vi "AdjustSpeaker.vi"(1 "Input Signal":refnum<vi>, 4 "Terminate":refnum<vi>, 5 "Peiker_Stepped Sweep Settings":T3={"Input Settings"={"IEPE min time to settle [s]"=0.0, "Responce Channel Settings"={"DSA response channel settings"={"coupling"=10045, "enable IEPE excitation"=FALSE, "IEPE current [mA]"=4.0}, "response channel info"={"sensor sensitivity"=200.0, "engineering units"=2, "dB reference"=2e-05, "custom label"="EU", "weighting filter"=0, "pregain"=0.0}, "AI response settings"={"response channel"="SOUNDACQ/ai1", "max value [V]"=10.0, "min value [V]"=-10.0, "terminal configuration"=-1}}, "Stimulus Channel Settings"={"AI stimulus settings"={"stimulus channel"="SOUNDACQ/ai0", "max value [V]"=10.0, "min value [V]"=-10.0, "terminal configuration"=-1}, "DSA stimulus channel settings"={"coupling"=10045, "enable IEPE excitation"=TRUE, "IEPE current [mA]"=4.0}, "stimulus channel info"={"sensor sensitivity"=11.4, "engineering units"=2, "dB reference"=2e-05, "custom label"="EU", "weighting filter"=0, "pregain"=0.0}}}, "Output Settings"={"AO source settings"={"excitation channel"="SOUNDACQ/ao0", "max value [V]"=10.0, "min value [V]"=-10.0, "terminal configuration"=-1}}} {"Output Settings"."AO source settings"."terminal configuration" items=["Default"=-1, "RSE"=10083, "Differential"=10106, "Pseudodifferential"=12529]; "Output Settings"."AO source settings"."min value [V]" format="%0.2f"; "Output Settings"."AO source settings"."max value [V]" format="%0.2f"; "Input Settings"."Stimulus Channel Settings"."stimulus channel info"."pregain" format="%.2f"; "Input Settings"."Stimulus Channel Settings"."stimulus channel info"."weighting filter" items=["Linear", "A-weighting", "B-weighting", "C-weighting", "ITU-R 468-4", "Dolby", "CCITT", "C-message", "Wb", "Wc", "Wd", "We", "Wf", "Wh", "Wj", "Wk", "Wm", "AES17 20 kHz lowpass", "AES17 40 kHz lowpass", "AES17 20 kHz highpass", "AES17 40 kHz highpass"]; "Input Settings"."Stimulus Channel Settings"."stimulus channel info"."dB reference" format="%^.1e"; "Input Settings"."Stimulus Channel Settings"."stimulus channel info"."engineering units" items=["custom..."=0, "V"=1, "A"=21, "C"=30, "pC"=31, "s"=32, "-"=29, "Pa"=2, "N"=20, "g"=3, "m/s^2"=4, "m/s"=5, "m"=6, "mm/s"=12, "mm"=13, "micron/s"=14, "micron"=15, "in/s^2"=7, "in/s"=8, "in"=9, "mil/s"=10, "mil"=11, "rad/s^2"=16, "rad/s"=17, "rad"=18, "deg/s^2"=26, "deg/s"=27, "deg"=28, "RPM"=22, "cycle/s^2"=23, "Hz"=24, "cycle"=25, "strain"=19]; "Input Settings"."Stimulus Channel Settings"."stimulus channel info"."sensor sensitivity" format="%#_5f"; "Input Settings"."Stimulus Channel Settings"."DSA stimulus channel settings"."IEPE current [mA]" format="%.1f"; "Input Settings"."Stimulus Channel Settings"."DSA stimulus channel settings"."coupling" items=["AC"=10045, "DC"=10050, "GND"=10066]; "Input Settings"."Stimulus Channel Settings"."AI stimulus settings"."terminal configuration" items=["Default"=-1, "RSE"=10083, "NRSE"=10078, "Differential"=10106, "Pseudodifferential"=12529]; "Input Settings"."Stimulus Channel Settings"."AI stimulus settings"."min value [V]" format="%.2f"; "Input Settings"."Stimulus Channel Settings"."AI stimulus settings"."max value [V]" format="%.2f"; "Input Settings"."Responce Channel Settings"."AI response settings"."terminal configuration" items=["Default"=-1, "RSE"=10083, "NRSE"=10078, "Differential"=10106, "Pseudodifferential"=12529]; "Input Settings"."Responce Channel Settings"."AI response settings"."min value [V]" format="%.2f"; "Input Settings"."Responce Channel Settings"."AI response settings"."max value [V]" format="%.2f"; "Input Settings"."Responce Channel Settings"."response channel info"."pregain" format="%.2f"; "Input Settings"."Responce Channel Settings"."response channel info"."weighting filter" items=["Linear", "A-weighting", "B-weighting", "C-weighting", "ITU-R 468-4", "Dolby", "CCITT", "C-message", "Wb", "Wc", "Wd", "We", "Wf", "Wh", "Wj", "Wk", "Wm", "AES17 20 kHz lowpass", "AES17 40 kHz lowpass", "AES17 20 kHz highpass", "AES17 40 kHz highpass"]; "Input Settings"."Responce Channel Settings"."response channel info"."dB reference" format="%^.1e"; "Input Settings"."Responce Channel Settings"."response channel info"."engineering units" items=["custom..."=0, "V"=1, "A"=21, "C"=30, "pC"=31, "s"=32, "-"=29, "Pa"=2, "N"=20, "g"=3, "m/s^2"=4, "m/s"=5, "m"=6, "mm/s"=12, "mm"=13, "micron/s"=14, "micron"=15, "in/s^2"=7, "in/s"=8, "in"=9, "mil/s"=10, "mil"=11, "rad/s^2"=16, "rad/s"=17, "rad"=18, "deg/s^2"=26, "deg/s"=27, "deg"=28, "RPM"=22, "cycle/s^2"=23, "Hz"=24, "cycle"=25, "strain"=19]; "Input Settings"."Responce Channel Settings"."response channel info"."sensor sensitivity" format="%#_5f"; "Input Settings"."Responce Channel Settings"."DSA response channel settings"."IEPE current [mA]" format="%.1f"; "Input Settings"."Responce Channel Settings"."DSA response channel settings"."coupling" items=["AC"=10045, "DC"=10050, "GND"=10066]; "Input Settings"."IEPE min time to settle [s]" format="%.1f"}, 6 "Fundamental Amplitude 2":refnum<vi>, 7 "CalSettings":T1={"SollPegel[dBSPL]"=114, "maxDeviationRef[dB]"=2.0, "maxDeviation[dB]"=2.0, "maxRuns"=20, "RefFrequency[Hz]"=1000, "Wait[ms]"=0} {"maxDeviation[dB]" format="%.2f"; "maxDeviationRef[dB]" format="%.2f"}, 8 "error in":errorcluster, 9 "integration time":T9={"integration time [s]"=0.015599999576807022, "integration cycles"=5} {"integration cycles" min=2; "integration time [s]" format="%.2p"}, 10 "settling time":T8={"settle time [s]"=0.015599999576807022, "settle cycles"=5} {"settle time [s]" format="%.2p"}, 11 "Frequency List":T2(array[cluster])) -> (0 "error out":errorcluster, 2 "magnitude":dbl[](array[numeric]), 3 "correctedFreqList":T2(array[cluster]))   [LabVIEW 2018]
uses:
  Peiker_Stepped Sweep Settings.ctl
  <vilib>/addons/_NISVFA/_Shared subVIs/Controls/svc_DSA Channel Settings.ctl
  <vilib>/addons/_NISVFA/_Shared subVIs/Controls/svc_Channel Info.ctl
  <vilib>/addons/_NISVFA/_Shared subVIs/Controls/svc_Engineering Units Text Ring.ctl
  <vilib>/addons/_NISVFA/_Shared subVIs/Controls/svc_Weighting Filter Text Ring.ctl
panel:
  out "error out 2":errorcluster
  out "max value":dbl
  out "min value":dbl
  out "RefValue":dbl
  in  "CalTablePath":path=path "D:/PRUEF/MIC_EOL_TS2016/Sourcecode/ProjectSourcecode/Config Files/calibrationResults.txt"
  out "runs":i32
  # "Input Parameters"
  # "Output Parameters"
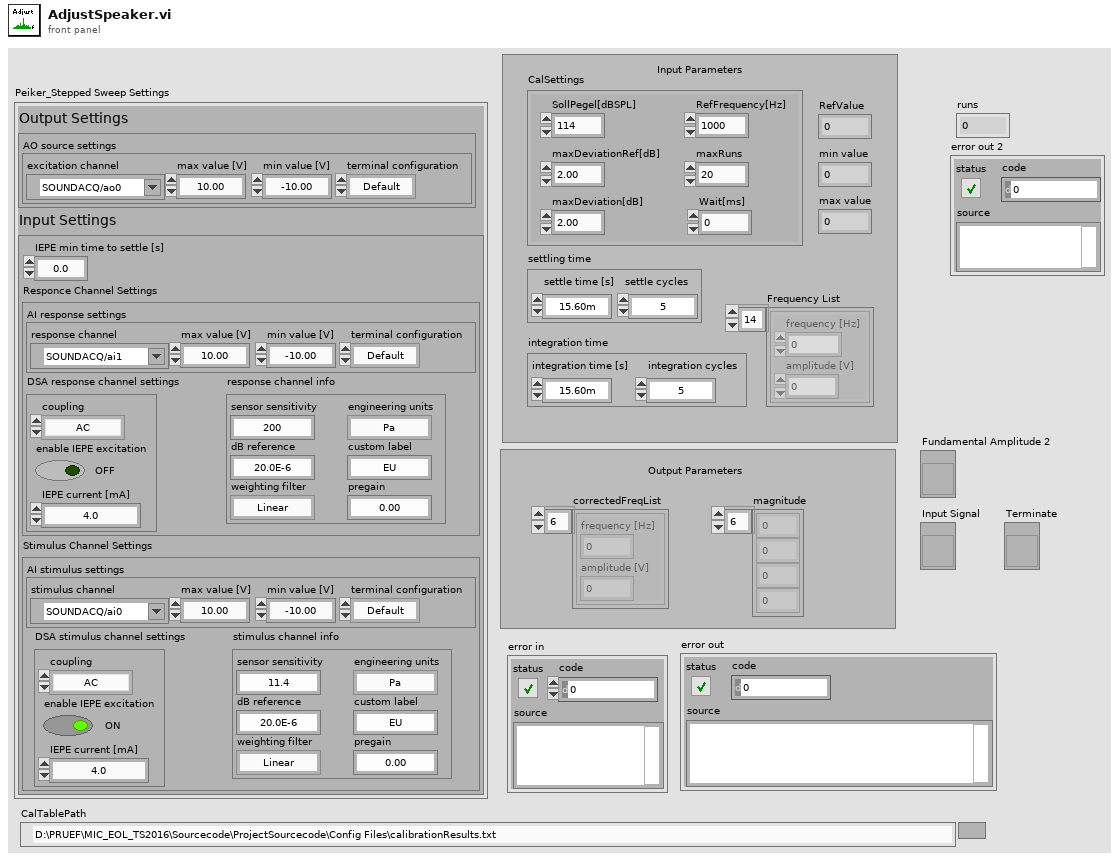
[diagram p1: front panel]
types:
  T1 = cluster{"SollPegel[dBSPL]":i32, "maxDeviationRef[dB]":dbl, "maxDeviation[dB]":dbl, "maxRuns":i32, "RefFrequency[Hz]":i32, "Wait[ms]":i32}
  T2 = cluster{"frequency [Hz]":dbl, "amplitude [V]":dbl}[]
  T3 = typedef "Peiker_Stepped Sweep Settings.ctl" = cluster{"Input Settings":cluster{"IEPE min time to settle [s]":dbl, "Responce Channel Settings":cluster{"DSA response channel settings":T4, "response channel info":T5, "AI response settings":cluster{"response channel":tag, "max value [V]":dbl, "min value [V]":dbl, "terminal configuration":i32}}, "Stimulus Channel Settings":cluster{"AI stimulus settings":cluster{"stimulus channel":tag, "max value [V]":dbl, "min value [V]":dbl, "terminal configuration":i32}, "DSA stimulus channel settings":T4, "stimulus channel info":T5}}, "Output Settings":cluster{"AO source settings":cluster{"excitation channel":tag, "max value [V]":dbl, "min value [V]":dbl, "terminal configuration":i32}}}
  T4 = typedef "svc_DSA Channel Settings.ctl" = cluster{"coupling":i32, "enable IEPE excitation":bool, "IEPE current [mA]":dbl}
  T5 = typedef "svc_Channel Info.ctl" = cluster{"sensor sensitivity":dbl, "engineering units":T6, "dB reference":dbl, "custom label":string, "weighting filter":T7, "pregain":dbl}
  T6 = typedef "svc_Engineering Units Text Ring.ctl" = u16
  T7 = typedef "svc_Weighting Filter Text Ring.ctl" = u16
  T8 = cluster{"settle time [s]":dbl, "settle cycles":i32}
  T9 = cluster{"integration time [s]":dbl, "integration cycles":i32}
  T10 = cluster{"frequency [Hz]":dbl[], "amplitude":dbl[]}
  T11 = cluster{"max value":dbl, "min value":dbl, "RefValue[dB]":dbl, "RefAmp[V]":dbl}
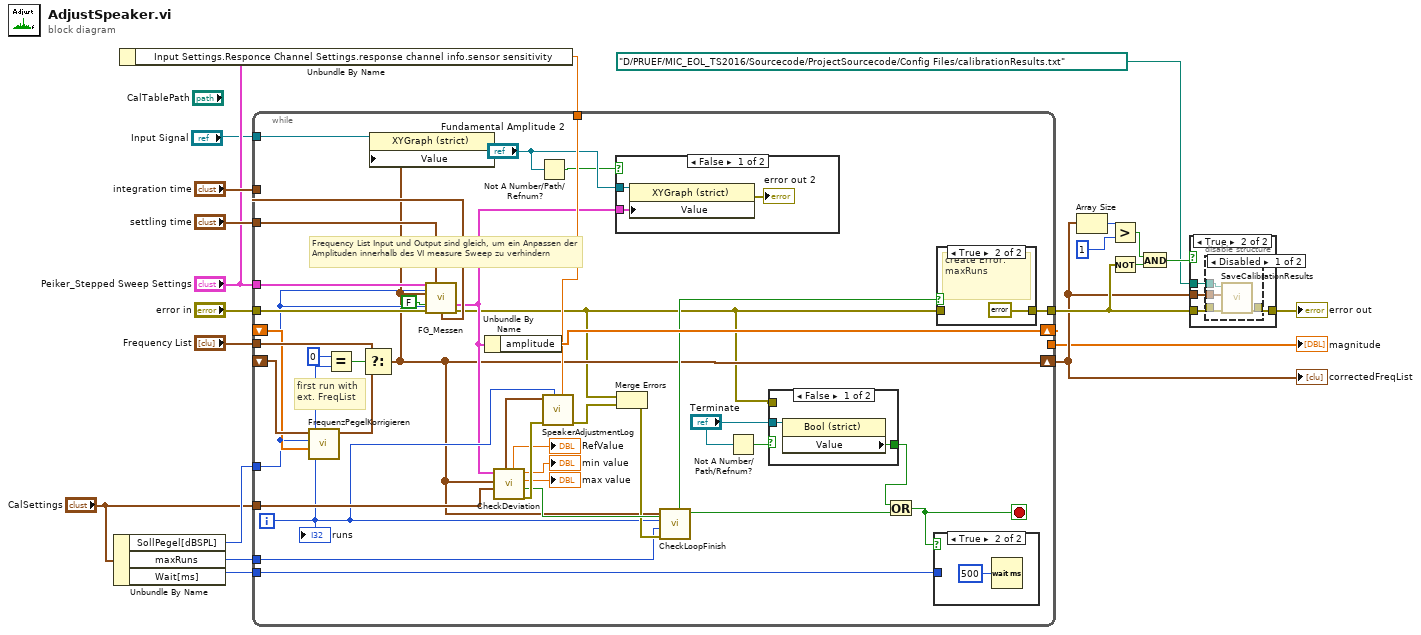
[diagram p0: block diagram]
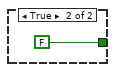
[diagram p4: hidden frame]
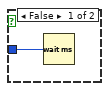
[diagram p6: hidden frame]
diagram:
  n1 = Unbundle By Name("CalSettings") -> ("SollPegel[dBSPL]"=w14:i32, "maxRuns"=w13:i32, "Wait[ms]"=w3:i32)
  n2 = Unbundle By Name("Peiker_Stepped Sweep Settings") -> ("Input Settings.Responce Channel Settings.response channel info.sensor sensitivity"=w4:dbl)
  n3 = while {
    tunnel: "Peiker_Stepped Sweep Settings" -> [w46]
    tunnel: "Frequency List" -> [w58]
    shift-right: [w28] -> w7
    shift-left: _ -> [w56]
    shift-right: [w48] -> _
    shift-left: _ -> [w55]
    tunnel: "error in" -> [w54]
    tunnel: "integration time" -> [w52]
    tunnel: "settling time" -> [w51]
    tunnel: w14 -> [w49]
    tunnel: [w50] -> w8
    tunnel: [w48] -> w5
    tunnel: w13 -> [w36]
    tunnel: "CalSettings" -> [w43]
    tunnel: w4 -> [w45]
    tunnel: w3 -> [w34]
    tunnel: "Input Signal" -> [w29]
    i -> [w35]
    stop <- w25 stop-if-true
    # "Frequency List Input und Output sind gleich, um ein Anpassen der Amplituden innerhalb des VI measure Sweep zu verhindern"
    # "first run with\next. FreqList"
    n4 = call "FrequenzPegelKorrigieren.vi"("gemessenerPegel"=w55, "SollPegel"=w49, "Frequency List"=w56) -> ("korrigierte Frequenzliste"=w57:T2)  [unwired: 8 in]
    n5 = Equal?(x=0, y=w35) -> (x = y?=w59:bool)
    n6 = Select(t=w58, s=w59, f=w57) -> (s? t:f=w28:T2)
    n7 = property class="XYGraph (strict)"(reference=w29, "Value"=w28) -> ()  [unwired: 1 in, 2 out]
    n8 = call "FG_Messen.vi"("Peiker_Stepped Sweep Settings"=w46, "settling time"=w51, "FrequencyList Output Level (dBSPL)"=w49, "frequency list Input"=w28, "true=mehrfach Messen"=FALSE, "error in (no error)"=w54, "FrequencyList Input Level (dBSPL)"=w49, "integration time"=w52) -> ("fundamental amplitude"=w32:T10, "error out"=w22:errorcluster)  [unwired: 1 in, 5 out]
    n9 = Unbundle By Name(w32) -> ("amplitude"=w48:dbl[])
    n10 = call "CheckDeviation.vi"("CalSettings"=w43, "Frequency List"=w28, "fundamental amplitude"=w32) -> ("error Out"=w47:errorcluster, "DeviationInRange"=w39:bool, "max value"=→"max value":dbl, "min value"=→"min value":dbl, "RefValue[dB]"=→"RefValue":dbl, "output cluster"=w44:T11)  [unwired: 3 in]
    n11 = Not A Number/Path/Refnum?(number/path/refnum="Fundamental Amplitude 2") -> (NaN/Path/Refnum?=w30:bool)
    n12 = call "SpeakerAdjustmentLog.vi"("SensorSens"=w45, "RunNo."=w35, "error in (no error)"=w47, "Input cluster"=w44) -> ("error IO"=w38:errorcluster)  [unwired: 7 in]
    n13 = case shown="False" w30 {
      tunnel: w32 -> [w66 _]
      tunnel: "Fundamental Amplitude 2" -> [w64 _]
      frame False {
        n14 = property class="XYGraph (strict)"(reference=w64, "Value"=w66) -> (error out=→"error out 2":errorcluster)  [unwired: 1 in, 1 out]
      }
      frame True {
      }
    }
    n15 = Merge Errors(w22, w38) -> (w37:errorcluster)
    n16 = call "CheckLoopFinish.vi"("Deviation"=w39, "error in"=w37, "maxRuns"=w36, "iCounter"=w35, "Frequency List"=w28) -> ("Stop Loop"=w26:bool, "maxRuns"=w33:bool)  [unwired: 5 in]
    n17 = Not A Number/Path/Refnum?(number/path/refnum="Terminate") -> (NaN/Path/Refnum?=w23:bool)
    n18 = case shown="False" w23 {
      tunnel: "Terminate" -> [w62 _]
      tunnel: [w61 FALSE ("Value")] -> w27
      tunnel: w22 -> [_ _]
      frame False {
        n19 = property class="Bool (strict)"(reference=w62) -> ("Value"=w61:bool)  [unwired: 1 in, 2 out]
      }
      frame True {
      }
    }
    n20 = Or(x=w27, y=w26) -> (x .or. y?=w25:bool)
    n21 = case shown="True" w25 {
      tunnel: w34 -> [w67 _]
      frame False {
        n22 = Wait (ms)(milliseconds to wait=w67) -> ()  [unwired: 1 out]
      }
      frame True {
        n23 = Wait (ms)(milliseconds to wait=u32 500) -> ()  [unwired: 1 out]
      }
    }
    n24 = case shown="True" w33 {
      tunnel: w22 -> [w69 _]
      tunnel: [w69 errorcluster {"status"=TRUE, "code"=5000, "source"="Anzahl der Abgleichdurchgänge zu hoch,\nPrüfen ob der Messaufbau korrekt ist."} ("error out 2")] -> w50
      frame False {
      }
      frame True {
        # "create Error:\nmaxRuns"
      }
    }
    "runs" <- w35
  }
  "correctedFreqList" <- w7
  "magnitude" <- w5
  n25 = Array Size(array=w7) -> (size(s)=w16:i32)
  n26 = Greater?(x=w16, y=1) -> (0:w11:bool)
  n27 = Not(x=w8) -> (.not. x?=w9:bool)
  n28 = And(x=w11, y=w9) -> (x .and. y?=w10:bool)
  n29 = case shown="True" w10 {
    tunnel: w8 -> [w71 w75]
    tunnel: [w71 w74] -> w6
    tunnel: w7 -> [_ w73]
    tunnel: path "D:/PRUEF/MIC_EOL_TS2016/Sourcecode/ProjectSourcecode/Config Files/calibrationResults.txt" ("CalTablePath") -> [_ w72]
    frame False {
    }
    frame True {
      n30 = disable-structure shown="Disabled" {
        disable-tunnel: w75 -> [w79 w80]
        disable-tunnel: [w78 w80] -> w74
        disable-tunnel: w73 -> [w77 _]
        disable-tunnel: w72 -> [w76 _]
        frame Disabled {
          n31 = call "SaveCalibrationResults.vi"("error in"=w79, "correctedFreqList"=w77, "file path calibration results"=w76) -> ("error out"=w78:errorcluster)  [unwired: 8 in]
        }
        frame Enabled {
        }
      }
    }
  }
  "error out" <- w6
